vi "FourFlippingCoins.vi"() -> ()   [LabVIEW 2015]
panel:
  out "Waveform Graph":i16[](graph)
  in  "Number of Trials":dbl
  out "Total Number of Heads":dbl
  out "Coin 4":bool
  out "Coin 3":bool
  out "Coin 2":bool
  out "Coin 1":bool
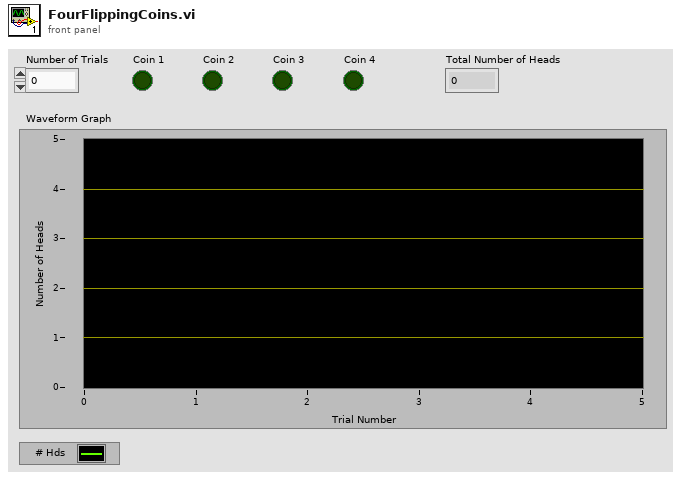
[diagram p1: front panel]
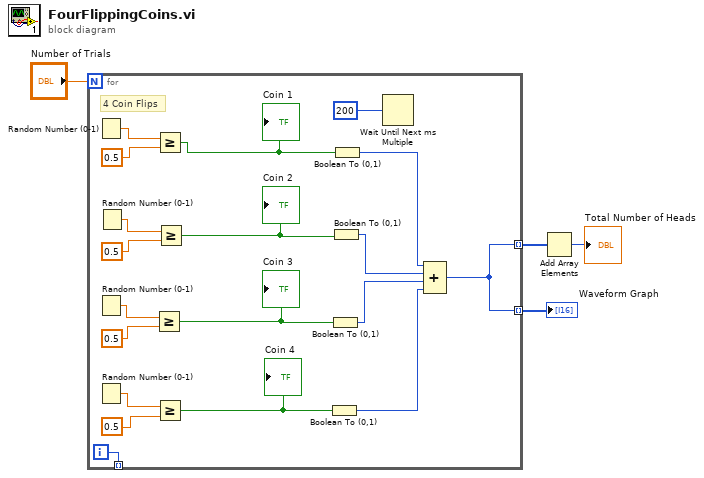
[diagram p0: block diagram]
diagram:
  n1 = for {
    N: "Number of Trials" -> [_]
    tunnel: [w7] -> _ mode=indexing
    tunnel: [w5] -> w2 mode=indexing
    tunnel: [w5] -> w1 mode=indexing
    i -> [w7]
    # "4 Coin Flips"
    n2 = Random Number (0-1)() -> (number: 0 to 1=w18:dbl)
    n3 = Random Number (0-1)() -> (number: 0 to 1=w13:dbl)
    n4 = Random Number (0-1)() -> (number: 0 to 1=w10:dbl)
    n5 = Random Number (0-1)() -> (number: 0 to 1=w15:dbl)
    n6 = Greater Or Equal?(x=w13, y=0.5) -> (x >= y?=w9:bool)
    "Coin 3" <- w9
    n7 = Greater Or Equal?(x=w18, y=0.5) -> (x >= y?=w17:bool)
    "Coin 1" <- w17
    n8 = Greater Or Equal?(x=w10, y=0.5) -> (x >= y?=w8:bool)
    "Coin 4" <- w8
    n9 = Greater Or Equal?(x=w15, y=0.5) -> (x >= y?=w11:bool)
    "Coin 2" <- w11
    n10 = Boolean To (0,1)(Boolean=w8) -> (0, 1=w20:i16)
    n11 = Boolean To (0,1)(Boolean=w9) -> (0, 1=w22:i16)
    n12 = Boolean To (0,1)(Boolean=w11) -> (0, 1=w23:i16)
    n13 = Boolean To (0,1)(Boolean=w17) -> (0, 1=w21:i16)
    n14 = Wait Until Next ms Multiple(millisecond multiple=200) -> ()  [unwired: 1 out]
    n15 = Compound Arithmetic op=ADD(w21, w23, w22, w20) -> (w5:i16)
  }
  "Waveform Graph" <- w1
  n16 = Add Array Elements(numeric array=w2) -> (sum=→"Total Number of Heads":i16)
